vi "Global 1.vi"() -> ()   [LabVIEW 2017]
panel:
  in  "Boolean":bool
  in  "Array":dbl[](array[numeric])
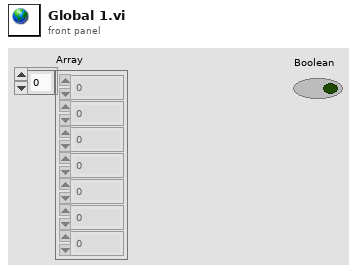
[diagram p1: front panel]
diagram:
